vi "TCPIP_SERVEUR_Array.vi"() -> ()   [LabVIEW 2018]
panel:
  out "Numeric":dbl
  out "Number of bytes":string
  out "Array":u8[](array[numeric])
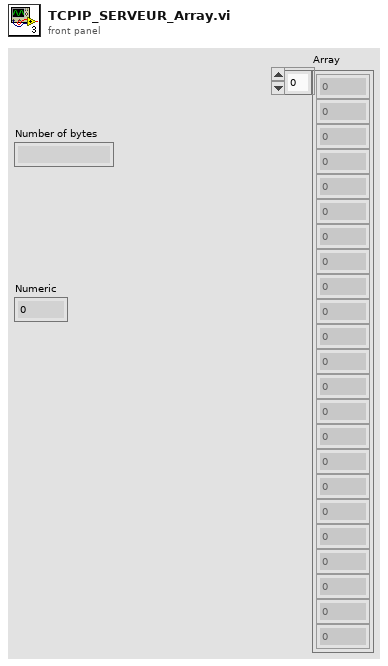
[diagram p1: front panel]
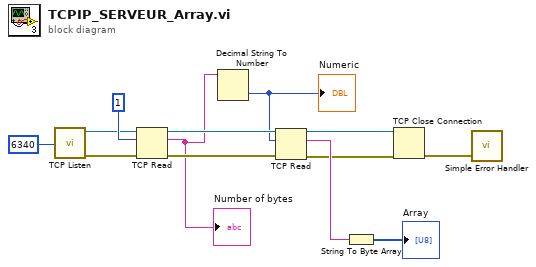
[diagram p0: block diagram]
diagram:
  n1 = call <vilib>:"TCP Listen.vi"("port"=6340) -> ("error out"=w4:errorcluster, "connection ID"=w5:refnum<k5>)  [unwired: 6 in, 3 out]
  n2 = TCP Read(connection ID=w5, bytes to read=1, error in (no error)=w4) -> (connection ID out=w11:refnum<k5>, data out=w8:string, error out=w10:errorcluster)  [unwired: 2 in]
  "Number of bytes" <- w8
  n3 = Decimal String To Number(string=w8) -> (number=w7:i32)  [unwired: 2 in, 1 out]
  "Numeric" <- w7
  n4 = TCP Read(connection ID=w11, bytes to read=w7, error in (no error)=w10) -> (connection ID out=w3:refnum<k5>, data out=w6:string, error out=w2:errorcluster)  [unwired: 2 in]
  n5 = String To Byte Array(string=w6) -> (unsigned byte array=→"Array":u8[])
  n6 = TCP Close Connection(connection ID=w3, error in (no error)=w2) -> (error out=w12:errorcluster)  [unwired: 1 in, 1 out]
  n7 = call <vilib>:"Simple Error Handler.vi"("error in (no error)"=w12) -> ()  [unwired: 4 in, 5 out]
